vi "Example Main Target.vi"() -> ()   [LabVIEW 2018]
uses:
  <vilib>/Platform/TimedLoop/XDataNode/timing_clust.ctl
  <vilib>/Platform/TimedLoop/XDataNode/nitl_modes.ctl
  <vilib>/Platform/TimedLoop/XDataNode/wakeup.ctl
  <vilib>/platform/TimedLoop/XDataNode/XDataNode.xnode
  <vilib>/Platform/TimedLoop/XDataNode/XDNodeRunTimeDep.lvlib
  COBRA Measurement and Filtering Library.lvlib
  <vilib>/ptbypt/NI_PtbyPt.lvlib
  <vilib>/Utility/Variable/NI_VariableUtilities.lvlib
panel:
  out "Target Stop":bool
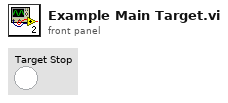
[diagram p1: front panel]
types:
  T1 = typedef "XDNodeRunTimeDep.lvlib/timing_clust.ctl" = cluster{"Expected End [f-1]":u64, "Actual End [f-1]":u64, "Finished Late? [f-1]":bool, "Expected End [i-1]":u64, "Actual End [i-1]":u64, "Finished Late? [i-1]":bool, "Expected Start [i]":u64, "Actual Start [i]":u64, "Expected Start [f]":u64, "Actual Start [f]":u64, "Source Name":string, "Structure Name":string, "Period":i64, "Deadline":i64, "Offset":i64, "Start":i64, "Priority":i32, "Timeout":i32, "Mode":T2, "Wakeup Reason":T3, "Error":errorcluster, "Source Type":string, "Secondary Source Type":string, "Global End Time":u64, "Global Start Time":u64, "Frame Duration":u64, "Iteration Duration":u64, "Assigned CPU":i32, "I/O Scan Engine Mode":u32}
  T2 = typedef "XDNodeRunTimeDep.lvlib/nitl_modes.ctl" = enum32{"No Change", "Process missed periods, maintain original phase", "Discard missed periods, maintain original phase", "Process missed periods, ignore original phase", "Discard missed periods, ignore original phase"}
  T3 = typedef "XDNodeRunTimeDep.lvlib/wakeup.ctl" = enum32{"Normal", "Aborted", "Asynchronous wakeup", "Timing source error", "Timed loop error", "Timeout"}
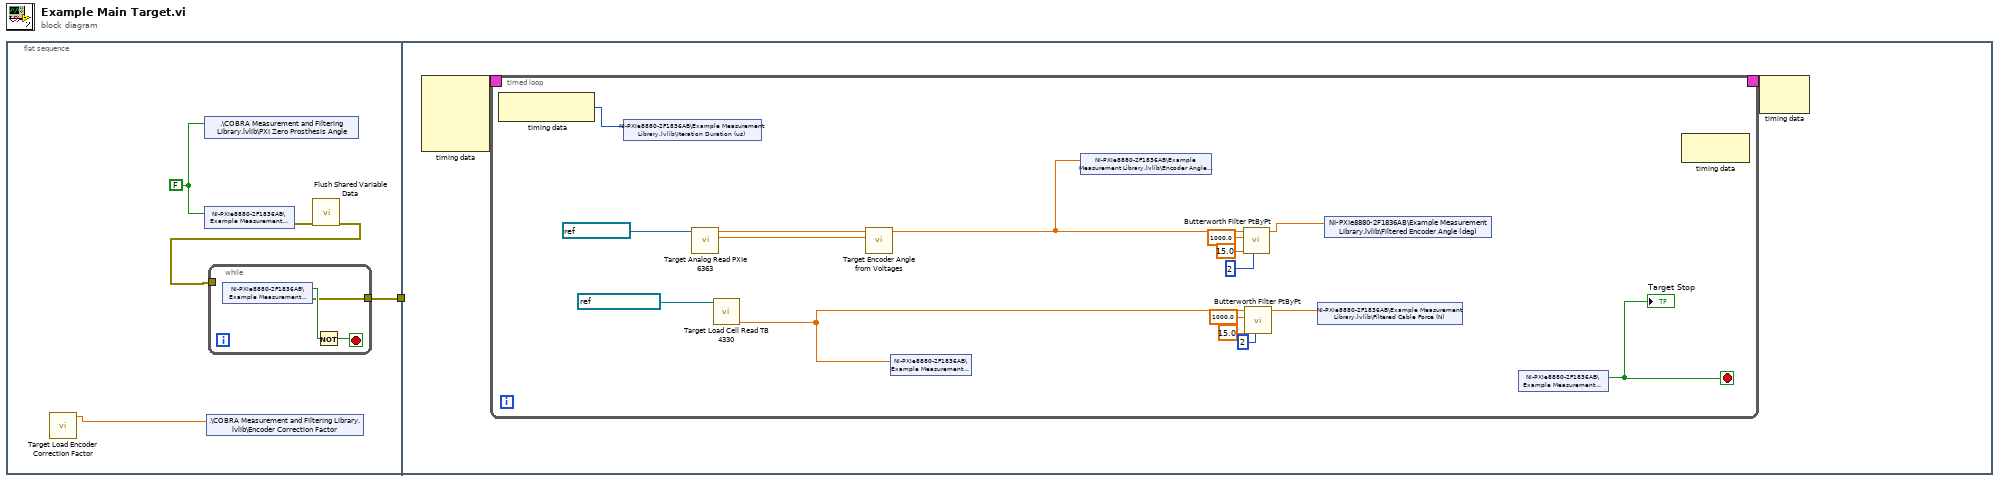
[diagram p0: block diagram]
diagram:
  n1 = flat-sequence {
    tunnel: [w3] -> w1
    tunnel: w1 -> [_]
    frame #0 {
      w6 = FALSE ("PXI Zero Prosthesis Angle")
      n2 = call "Target Load Encoder Correction Factor.vi"() -> ("Encoder Correction Factor"=w2:dbl)  [unwired: 11 in]
      n3 = shared-variable "NI-PXIe8880-2F1836AB\\Example Measurement Library.lvlib\\Target Stop"(w6) -> (error out=w5:errorcluster)  [unwired: 1 in]
      n4 = shared-variable ".\\COBRA Measurement and Filtering Library.lvlib\\PXI Zero Prosthesis Angle"(w6) -> ()  [unwired: 1 in, 1 out]
      n5 = shared-variable ".\\COBRA Measurement and Filtering Library.lvlib\\Encoder Correction Factor"(w2) -> ()  [unwired: 1 in, 1 out]
      n6 = call <vilib>:"Flush Shared Variable Data.vi"("error in (no error)"=w5) -> ("error out"=w4:errorcluster)  [unwired: 10 in]
      n7 = while {
        tunnel: w4 -> [_]
        tunnel: [w7] -> w3
        stop <- w9 stop-if-true
        n8 = shared-variable "NI-PXIe8880-2F1836AB\\Example Measurement Library.lvlib\\Target Stop"() -> (w8:bool, error out=w7:errorcluster)  [unwired: 1 in]
        n9 = Not(x=w8) -> (.not. x?=w9:bool)
      }
    }
    frame #1 {
      n10 = node-c288() -> (w11:T1)  [unwired: 4 in]
      n11 = timed-loop {
        timing: w11 -> [_]
        timing-out: [_] -> w10
        stop <- w24 stop-if-true
        n12 = node-c288() -> (w23:i64)  [unwired: 1 in]
        n13 = shared-variable "NI-PXIe8880-2F1836AB\\Example Measurement Library.lvlib\\Iteration Duration (us)"(w23) -> ()  [unwired: 1 in, 1 out]
        n14 = call "Target Analog Read PXIe 6363.vi"("task/channels in"=refnum<k21> "PXIe-6363") -> ("Encoder Voltage B"=w25:dbl, "Encoder Voltage A"=w26:dbl)  [unwired: 7 in, 2 out]
        n15 = call "Target Load Cell Read TB 4330.vi"("task/channels in"=refnum<k21> "Futek 844206") -> ("Cable Force (N)"=w21:dbl)  [unwired: 10 in]
        n16 = call "Target Encoder Angle from Voltages.vi"("Encoder Voltage B (V)"=w25, "Encoder Voltage A (V)"=w26) -> ("Encoder Angle (deg)"=w19:dbl)  [unwired: 9 in]
        n17 = shared-variable "NI-PXIe8880-2F1836AB\\Example Measurement Library.lvlib\\Force (N)"(w21) -> ()  [unwired: 1 in, 1 out]
        n18 = shared-variable "NI-PXIe8880-2F1836AB\\Example Measurement Library.lvlib\\Encoder Angle (deg)"(w19) -> ()  [unwired: 1 in, 1 out]
        n19 = call <vilib>:"Butterworth Filter PtByPt.vi"("order"=2, "low cutoff freq: fl"=15.0, "sampling freq: fs"=1000.0, "x"=w19) -> ("Filtered x"=w13:dbl)  [unwired: 5 in, 1 out]
        n20 = call <vilib>:"Butterworth Filter PtByPt.vi"("order"=2, "low cutoff freq: fl"=15.0, "sampling freq: fs"=1000.0, "x"=w21) -> ("Filtered x"=w12:dbl)  [unwired: 5 in, 1 out]
        n21 = shared-variable "NI-PXIe8880-2F1836AB\\Example Measurement Library.lvlib\\Filtered Cable Force (N)"(w12) -> ()  [unwired: 1 in, 1 out]
        n22 = shared-variable "NI-PXIe8880-2F1836AB\\Example Measurement Library.lvlib\\Filtered Encoder Angle (deg)"(w13) -> ()  [unwired: 1 in, 1 out]
        n23 = shared-variable "NI-PXIe8880-2F1836AB\\Example Measurement Library.lvlib\\Target Stop"() -> (w24:bool)  [unwired: 1 in, 1 out]
        "Target Stop" <- w24
        n24 = node-c288() -> ()  [unwired: 1 in, 1 out]
      }
      n25 = node-c288(w10) -> ()  [unwired: 1 out]
    }
  }
